vi "UPRcontroller_v00_basedonlsmv66.vi"() -> ()   [LabVIEW 2015] (continued)
                          n5180 = Unbundle By Name(w2176) -> ("dt"=w2175:dbl, "Y"=w2178:dbl[])
                          n5181 = Reciprocal(x=w2175) -> (1/x=w2174:dbl)
                          n5182 = Array Size(array=w2178) -> (size(s)=w2177:i32)
                          n5183 = Round To Nearest(number=w2174) -> (nearest integer value=w2173:dbl)
                        }
                        frame 1, Default {
                        }
                      }
                    }
                    n5184 = Index Array(array=w2152, index=0) -> (element=w2154:i32)
                    n5185 = Index Array(array=w2140, index=0) -> (element=w2139:dbl)
                    n5186 = for {
                      tunnel: w2151 -> [w2159] mode=indexing
                      tunnel: [w2157] -> w2138 mode=indexing
                      tunnel: w2154 -> [w2156]
                      n5187 = Unbundle By Name(w2159) -> ("DOtab"=w2158:dbl)
                      n5188 = case shown="1" w2158 {
                        tunnel: w2159 -> [w2162 w2164]
                        tunnel: w2156 -> [w2161 _]
                        tunnel: [w2160 w2163] -> w2157
                        frame 0, Default {
                          n5189 = call "simple digital from wf params.vi"("waveform params"=w2162, "number of samples"=w2161) -> ("digital waveform"=w2160:digitalwaveform)
                        }
                        frame 1 {
                          n5190 = call "matlabDOwffromparam.vi"("waveform params"=w2164) -> ("digital waveform"=w2163:digitalwaveform)
                        }
                      }
                    }
                    n5191 = property on="refwf" class="Ring (strict)"() -> ("RingText.Text"=w2142:string)  [unwired: 2 in, 2 out]
                    n5192 = call "correctwaveformsizetemp.vi"("new sampling frequency (Hz)"=w2139, "start"=FALSE, "reference waveforms to"=w2142, "Analog waveforms in"=w2137, "stop"=FALSE, "Digital waveforms in"=w2138) -> ("analog wf out"=w2136:waveform(dbl)[], "Digital wf out"=w2135:digitalwaveform[], "measpoints"=w2133:i32)
                    n5193 = local read "wavdet"() -> (w2134:bool)
                    n5194 = case shown="True" w2134 {
                      tunnel: w2133 -> [_ w2155]
                      frame False {
                      }
                      frame True {
                        n5195 = local write "# of frames"(w2155) -> ()
                      }
                    }
                    n5196 = local write "Analog Lines Plot"(w2136) -> ()
                    n5197 = local write "Digital Lines Plot"(w2135) -> ()
                    n5198 = call "GetNumCamFramesv2.vi"("Digital Waveform Graph"=w2135) -> ("Numeric"=w2147:i32)  [unwired: 10 in]
                    n5199 = call "waveformsAObuffer.vi"("AO wf in"=w2136, "command"="set") -> ()  [unwired: 1 out]
                    n5200 = call "waveformsDObuffer.vi"("DO wf in"=w2135, "command"="set") -> ()  [unwired: 1 out]
                    n5201 = local write "Total Camera Frames"(w2147) -> ()
                  }
                  frame #4 {
                    n5202 = local read "AO channels"() -> (w2188:u32)
                    n5203 = call "2pparameters.vi"("command"="get") -> ("params out"=w2190:T12)  [unwired: 1 in]
                    n5204 = Unbundle By Name(w2190) -> ("aAO"=w2189:u32[])
                    n5205 = Search 1D Array(1D array=w2189, element=w2188) -> (index of element=w2192:i32)  [unwired: 1 in]
                    n5206 = Equal?(x=w2192, y=-1.0) -> (x = y?=w2193:bool)
                    n5207 = case shown="False" w2193 {
                      tunnel: w2192 -> [w2218 _]
                      frame False {
                        n5208 = call "waveformparamsv2.vi"("command"="get") -> ("Params out"=w2201:T17)  [unwired: 4 in, 2 out]
                        n5209 = Unbundle By Name(w2201) -> ("AO parameters"=w2200:T18)
                        n5210 = Index Array(array=w2200, index=w2218) -> (element=w2217:T19)
                        n5211 = Unbundle By Name(w2217) -> ("AOtab"=w2198:dbl, "Repeats"=w2216:dbl, "Cycles"=w2215:dbl, "Start amplitude (V)"=w2214:dbl, "Baseline (V)"=w2213:dbl, "Step size (V)"=w2212:dbl, "DC (%)"=w2211:dbl, "Sampling frequency (Hz)"=w2210:dbl, "Period (ms)"=w2209:dbl, "Offset (V)"=w2208:dbl, "Amplitude (V)"=w2207:dbl, "Frequency"=w2206:dbl, "Tri Repeats"=w2205:dbl, "phase shift (ms)"=w2204:dbl, "Pulses"=w2203:dbl, "Tri phase"=w2199:dbl, "padding value"=w2195:dbl, "Matlab wave file"=w2196:path)
                        n5212 = To Unsigned Long Integer(number=w2198) -> (unsigned 32bit integer=w2197:u32)
                        n5213 = local write "Build analog waveform tabs"(w2197) -> ()
                        n5214 = local write "Matlab waveform path"(w2196) -> ()
                        n5215 = local write "phase shift (ms)"(w2204) -> ()
                        n5216 = local write "Repeats"(w2216) -> ()
                        n5217 = local write "Cycles"(w2215) -> ()
                        n5218 = local write "Amplitude (V)"(w2207) -> ()
                        n5219 = local write "Matlab padding value"(w2195) -> ()
                        n5220 = local write "Tri padding value"(w2195) -> ()
                        n5221 = local write "Start amplitude (V)"(w2214) -> ()
                        n5222 = local write "Tri Phase (s)"(w2199) -> ()
                        n5223 = local write "Period (ms)"(w2209) -> ()
                        n5224 = local write "Tri Repeats"(w2205) -> ()
                        n5225 = local write "Offset (V)"(w2208) -> ()
                        n5226 = local write "Frequency"(w2206) -> ()
                        n5227 = local write "Pulses"(w2203) -> ()
                        n5228 = local write "padding value"(w2195) -> ()
                        n5229 = local write "Sampling rate \ncurrent wf"(w2210) -> ()
                        n5230 = local write "Baseline (V)"(w2213) -> ()
                        n5231 = local write "Step size (V)"(w2212) -> ()
                        n5232 = local write "DC (%)"(w2211) -> ()
                      }
                      frame True {
                      }
                    }
                  }
                  frame #5 {
                    n5233 = local read "DO channels"() -> (w2221:u16)
                    n5234 = call "2pparameters.vi"("command"="get") -> ("params out"=w2223:T12)  [unwired: 1 in]
                    n5235 = Unbundle By Name(w2223) -> ("aDO"=w2222:u32[])
                    n5236 = Search 1D Array(1D array=w2222, element=w2221) -> (index of element=w2220:i32)  [unwired: 1 in]
                    n5237 = Equal?(x=w2220, y=-1.0) -> (x = y?=w2219:bool)
                    n5238 = case shown="False" w2219 {
                      tunnel: w2220 -> [w2238 _]
                      frame False {
                        n5239 = call "waveformparamsv2.vi"("command"="get") -> ("Params out"=w2232:T17)  [unwired: 4 in, 2 out]
                        n5240 = Unbundle By Name(w2232) -> ("DO parameters"=w2230:T20)
                        n5241 = Index Array(array=w2230, index=w2238) -> (element=w2237:T21)
                        n5242 = Unbundle By Name(w2237) -> ("Digital DC (%)"=w2236:dbl, "Digital phase"=w2235:dbl, "Digital Freq (Hz)"=w2234:dbl, "Sampling frequency (Hz)"=w2233:dbl, "Digital time offset (s)"=w2229:dbl, "padding value"=w2228:dbl, "matlab wave file"=w2227:path, "DOtab"=w2226:dbl)
                        n5243 = local write "Build digital waveform tabs"(w2226) -> ()
                        n5244 = local write "Digital DC (%)"(w2236) -> ()
                        n5245 = local write "Matlab waveform path DO"(w2227) -> ()
                        n5246 = local write "Sampling rate \ncurrent wf"(w2233) -> ()
                        n5247 = local write "Digital time offset (s)"(w2229) -> ()
                        n5248 = local write "Matlab padding value DO"(w2228) -> ()
                        n5249 = local write "Digital padding value"(w2228) -> ()
                        n5250 = local write "Digital Freq (Hz)"(w2234) -> ()
                        n5251 = local write "Digital phase (s)"(w2235) -> ()
                      }
                      frame True {
                      }
                    }
                  }
                  frame #6 {
                    n5252 = local read "finite samples"() -> (w2240:bool)
                    n5253 = local read "continuous"() -> (w2241:bool)
                    n5254 = local read "wavdet"() -> (w2242:bool)
                    n5255 = call "2pparameters.vi"("command"="get") -> ("params out"=w2245:T12)  [unwired: 1 in]
                    n5256 = Bundle By Name(cluster=w2245, "finite"=w2240, "cont"=w2241, "wavdet"=w2242) -> (w2243:T12)
                    n5257 = property on="Update settings" class="Bool (strict)"("Val(Sgnl)"=FALSE ("Value (Signaling)")) -> ()  [unwired: 2 in, 2 out]
                    n5258 = call "2pparameters.vi"("Params in"=w2243, "command"="set") -> ()  [unwired: 1 out]
                  }
                }
              }
            }
          }
          event "Digital phase (s)", "Digital DC (%)", "Digital Freq (Hz)", "Digital padding value", "Digital time offset (s)": Value Change {
            n5259 = event-data() -> ()  [unwired: 1 in, 6 out]
            n5260 = local write "not loadedDO"(TRUE ("not loadedDO")) -> ()
          }
          event "Matlab padding value DO", "Matlab waveform path DO": Value Change {
            n5261 = event-data() -> ()  [unwired: 1 in, 6 out]
            n5262 = local write "not loadedDOml"(TRUE ("not loadedDO")) -> ()
          }
          event "phase shift (ms)", "Pulses", "Baseline (V)", "Step size (V)", "Start amplitude (V)", "Period (ms)", "DC (%)", "Cycles", "Repeats", "padding value": Value Change {
            n5263 = event-data() -> ()  [unwired: 1 in, 6 out]
            n5264 = local write "not loaded"(TRUE ("not loaded")) -> ()
          }
          event "Tri Repeats", "Amplitude (V)", "Offset (V)", "Frequency", "Tri Phase (s)", "Tri padding value": Value Change {
            n5265 = event-data() -> ()  [unwired: 1 in, 6 out]
            n5266 = local write "not loadedtri"(TRUE ("not loadedtri")) -> ()
          }
          event "Matlab waveform path", "Matlab padding value": Value Change {
            n5267 = event-data() -> ()  [unwired: 1 in, 6 out]
            n5268 = local write "not loadedml"(TRUE ("not loadedml")) -> ()
          }
          event "Exit": Value Change {
            n5269 = event-data() -> ("NewVal"=w2252:bool)  [unwired: 1 in]
          }
        }
        n5270 = Wait (ms)(milliseconds to wait=u32 50) -> ()  [unwired: 1 out]
      }
    }
    frame #3 {
      w6916 = FALSE ("Value (Signaling)")
      n5271 = property on="Start" class="Bool (strict)"("Val(Sgnl)"=w6916) -> ()  [unwired: 2 in, 2 out]
      n5272 = property on="Exit" class="Bool (strict)"("Val(Sgnl)"=w6916) -> ()  [unwired: 2 in, 2 out]
      n5273 = property on="Stop" class="Bool (strict)"("Val(Sgnl)"=w6916) -> ()  [unwired: 2 in, 2 out]
      n5274 = flat-sequence {
        frame #0 {
          n5275 = disable-structure shown="Disabled" {
            frame Disabled {
              w6917 = u16 1 items=["OD 0"=1, "OD 0.5"=2, "OD 1"=3, "OD 2"=4, "OD 3"=5, "OD 4"=6] ("New ODfilt")
              n5276 = local read "ODfilt"() -> (w6918:u16)
              n5277 = call "filterwheelcontrol_nothorlabslib.vi"("Current OD filt"=w6918, "New ODfilt"=w6917) -> ()  [unwired: 1 in]
            }
            frame Enabled {
            }
          }
        }
        frame #1 {
          n5278 = Wait (ms)(milliseconds to wait=u32 1000) -> ()  [unwired: 1 out]
        }
      }
    }
  }
